vi "Get Persistence.vi"(8 "error in (no error)":errorcluster, 11 "SigMan in":refnum<class "SignalManager.lvclass">) -> (0 "error out":errorcluster, 2 "persist":bool[](array[boolean]), 3 "SigMan out":refnum<class "SignalManager.lvclass">)   [LabVIEW 2020, in "SignalManager.lvclass"]
uses:
  SignalManager.lvclass
  SignalManager.lvclass/SignalManager.ctl
  Channel/Channel.lvclass/Channel.ctl
  Channel/Read Persist.vi
  Channel/Read Destination.vi
  Channel/Channel.lvclass
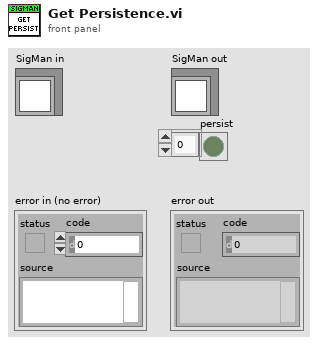
[diagram p1: front panel]
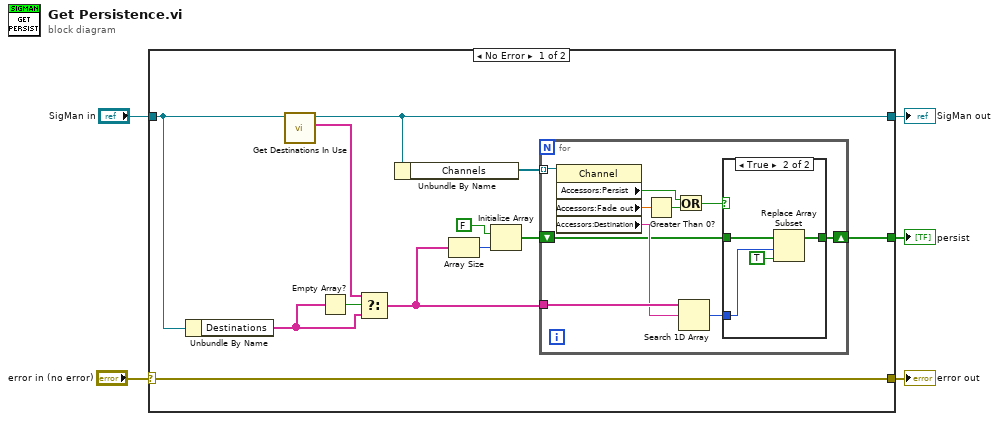
[diagram p0: block diagram]
diagram:
  n1 = case shown="No Error" "error in (no error)" {
    selector: "error in (no error)" -> [w6 w34]
    tunnel: [w6 w34] -> w4
    tunnel: [w13 w33] -> w2
    tunnel: "SigMan in" -> [w17 w33]
    tunnel: [w7 _] -> w1
    frame No Error {
      n2 = Unbundle By Name(w17) -> ("Destinations"=w14:string[])
      n3 = call "Get Destinations In Use.vi"("SigMan in"=w17) -> ("Destinations in use"=w15:string[], "SigMan out"=w13:refnum<class "SignalManager.lvclass">)  [unwired: 8 in, 1 out]
      n4 = Empty Array?(array=w14) -> (empty?=w16:bool)
      n5 = Select(t=w15, s=w16, f=w14) -> (s? t:f=w10:string[])
      n6 = Unbundle By Name(w13) -> ("Channels"=w12:refnum<class "Channel.lvclass">[])
      n7 = Array Size(array=w10) -> (size(s)=w11:i32)
      n8 = Initialize Array(FALSE, w11) -> (w8:bool[])
      n9 = for {
        tunnel: w12 -> [w27] mode=indexing
        tunnel: w10 -> [w26]
        shift-right: [w23] -> w7
        shift-left: w8 -> [w24]
        n10 = property class="Channel"(reference=w27) -> ("Accessors:Persist"=w19:bool, "Accessors:Fade out"=w21:dbl, "Accessors:Destination"=w25:string)  [unwired: 1 in, 2 out]
        n11 = Greater Than 0?(x=w21) -> (x > 0?=w20:bool)
        n12 = Or(x=w19, y=w20) -> (x .or. y?=w18:bool)
        n13 = Search 1D Array(1D array=w26, element=w25) -> (index of element=w22:i32)  [unwired: 1 in]
        n14 = case shown="True" w18 {
          tunnel: w24 -> [w28 w31]
          tunnel: [w28 w32] -> w23
          tunnel: w22 -> [_ w30]
          frame False {
          }
          frame True {
            n15 = Replace Array Subset(array=w31, new element=TRUE ("new element/subarray"), index=w30) -> (w32:bool[])
          }
        }
      }
    }
    frame Error {
    }
  }
  "error out" <- w4
  "SigMan out" <- w2
  "persist" <- w1
